vi "Error Debugger.vi"(8 "error in (no error)":errorcluster, 10 "Numeric":i32) -> (0 "error out":errorcluster)   [LabVIEW 2015]
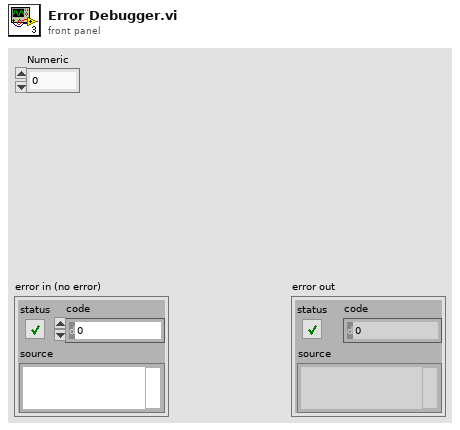
[diagram p1: front panel]
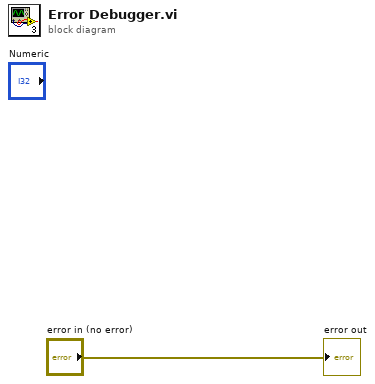
[diagram p0: block diagram]
diagram:
  "error out" <- "error in (no error)"
